vi "Translator.Test.vi"() -> ()   [LabVIEW 2019, in "Tools.lvlib"]
uses:
  Tools.lvlib
  Modules/Test_Panel/subVI/Test_Panel.UutTable/Test_Panel.UutTable.DisplayMode.ctl
  controls/buttons/Close.ctl
  Modules/Test_Panel/subVI/Test_Panel.HeaderData.ctl
panel:
  out "Test_Panel.HeaderData":T1
  in  "Close Button":T2 caption="Button"
  in  "results table view":T3 items=["all steps", "only teststeps", "teststeps w/seqcalls"]
  out "UUT SN":string="-" caption=")    SN:"
  out "Socket number":string="0" caption="Aktywny UUT (gniazdo:"
  out "Product":string="-" caption="Produkt:"
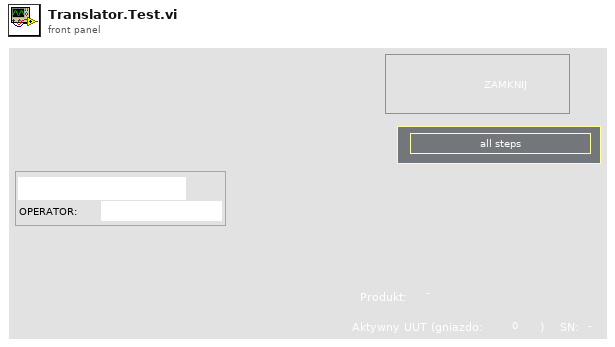
[diagram p1: front panel]
types:
  T1 = typedef "Test_Panel.HeaderData.ctl" = cluster{"operator":string, "time":string}
  T2 = typedef "Tools.lvlib/Close.ctl" = bool
  T3 = typedef "Test_Panel.UutTable.DisplayMode.ctl" = u16
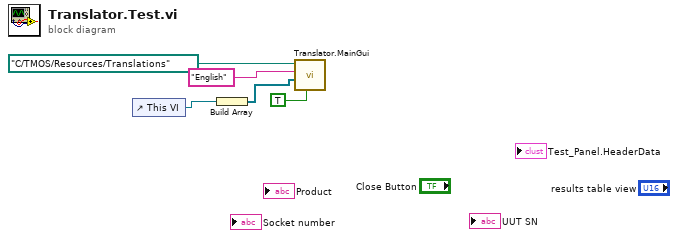
[diagram p0: block diagram]
diagram:
  n1 = control-ref of="This VI"() -> (w2:refnum<vi>)
  n2 = Build Array(w2) -> (w1:refnum<vi>[])
  n3 = call "Translator.MainGui.vi"("~Do not save font? (F)"=TRUE, "VI ref in [ ]"=w1, "~Language in use"="English", "~Translation folder"=path "C:/TMOS/Resources/Translations") -> ()  [unwired: 4 in, 4 out]
